vi "generate_temp_directory.vi"(8 "error in (no error)":errorcluster, 11 "configuration":T1) -> (0 "error out":errorcluster, 3 "temp_dir":path)   [LabVIEW 2015, in "lv-bin.lvlib" / "v1.lvlib"]
uses:
  v1.lvlib
  _controls/temp_dir_config.ctl
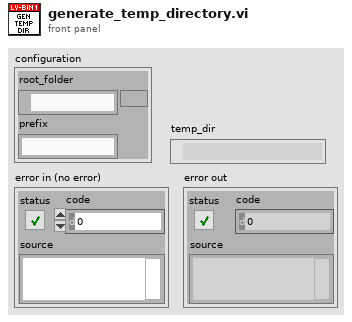
[diagram p1: front panel]
types:
  T1 = typedef "lv-bin.lvlib/v1.lvlib/temp_dir_config.ctl" = cluster{"root_folder":path, "prefix":string}
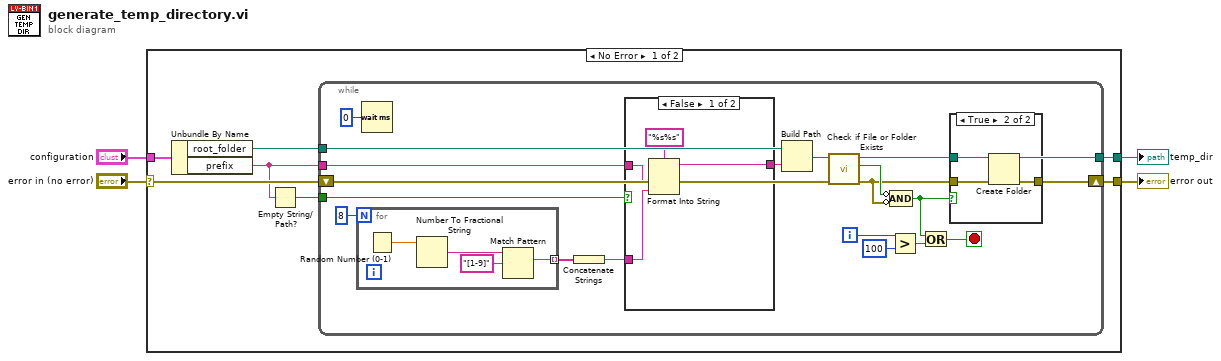
[diagram p0: block diagram]
diagram:
  n1 = case shown="No Error" "error in (no error)" {
    selector: "error in (no error)" -> [w11 w44]
    tunnel: [w7 _] -> w3
    tunnel: [w6 w44] -> w2
    tunnel: "configuration" -> [w5 _]
    frame No Error {
      n2 = Unbundle By Name(w5) -> ("root_folder"=w10:path, "prefix"=w9:string)
      n3 = Empty String/Path?(string/path=w9) -> (empty?=w8:bool)
      n4 = while {
        tunnel: w9 -> [w27]
        tunnel: w10 -> [w28]
        tunnel: w8 -> [w26]
        shift-right: [w12] -> w6
        shift-left: w11 -> [w15]
        tunnel: [w13] -> w7
        i -> [w20]
        stop <- w21 stop-if-true
        n5 = for {
          N: 8 -> [_]
          tunnel: [w40] -> w30 mode=indexing
          n6 = Random Number (0-1)() -> (number: 0 to 1=w43:dbl)
          n7 = Number To Fractional String(number=w43) -> (F-format string=w42:string)  [unwired: 3 in]
          n8 = Match Pattern(string=w42, regular expression="[1-9]") -> (match substring=w40:string)  [unwired: 1 in, 3 out]
        }
        n9 = Wait (ms)(milliseconds to wait=u32 0) -> ()  [unwired: 1 out]
        n10 = Concatenate Strings(w30) -> (w25:string)
        n11 = case shown="False" w26 {
          tunnel: w27 -> [w36 _]
          tunnel: w25 -> [w35 w39]
          tunnel: [w37 w39] -> w24
          frame False {
            n12 = Format Into String(format string="%s%s", w36, w35) -> (resulting string=w37:string)  [unwired: 2 in, 1 out]
          }
          frame True {
          }
        }
        n13 = Build Path(base path=w28, name or relative path=w24) -> (appended path=w23:path)
        n14 = call <vilib>:"Check if File or Folder Exists.vi"("error in (no error)"=w15, "path"=w23) -> ("error out"=w14:errorcluster, "file or folder exists?"=w22:bool, "dup path"=w13:path)  [unwired: 7 in]
        n15 = Compound Arithmetic op=AND(invert w22, invert w14) -> (w17:bool)
        n16 = Greater?(x=w20, y=100) -> (0:w18:bool)
        n17 = Or(x=w17, y=w18) -> (x .or. y?=w21:bool)
        n18 = case shown="True" w17 {
          tunnel: w13 -> [_ w34]
          tunnel: w14 -> [w31 w33]
          tunnel: [w31 w32] -> w12
          frame False {
          }
          frame True {
            n19 = Create Folder(path (use dialog)=w34, error in=w33) -> (error out=w32:errorcluster)  [unwired: 1 in, 2 out]
          }
        }
      }
    }
    frame Error {
    }
  }
  "error out" <- w2
  "temp_dir" <- w3
